vi "GA Get Gear Event.vi"(7 "pStartPara1":dbl, 8 "error in (no error)":errorcluster caption="错误输入（无错误）", 9 "pStartPara0":dbl, 10 "pEvent":i16, 11 "nAxisNum":i16) -> (0 "error out":errorcluster caption="错误输出", 1 "pStartPara0 out":dbl, 2 "pEvent out":i16, 3 "function return":i32, 5 "pStartPara1 out":dbl)   [LabVIEW 2015, in "GAS.lvlib"]
doc: "extern \"C\" __declspec(dllimport) int GA_GetGearEvent(short nAxisNum,short *pEvent,double *pStartPara0,double *pStartPara1);"
uses:
  <userlib>/BP_GAS/GAS.lvlib
  <userlib>/BP_GAS/GAS.dll
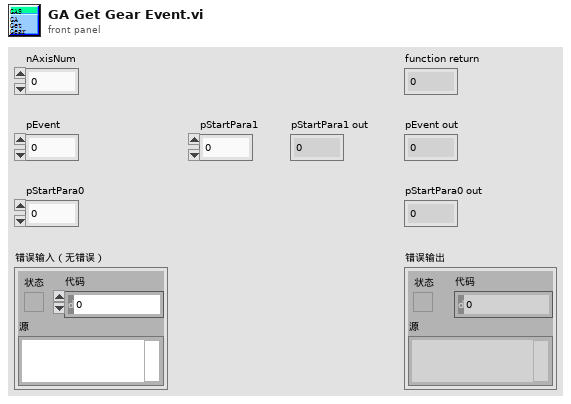
[diagram p1: front panel]
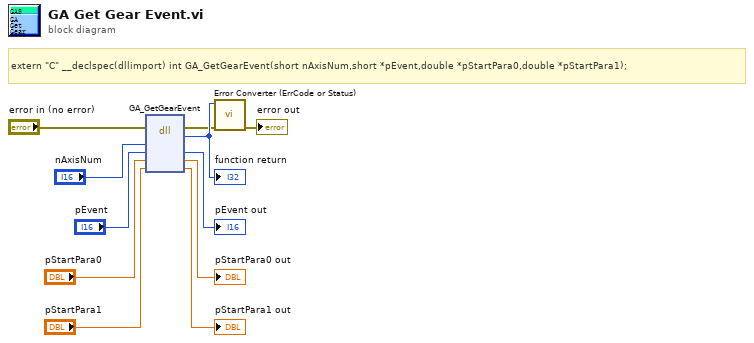
[diagram p0: block diagram]
diagram:
  # "extern \"C\" __declspec(dllimport) int GA_GetGearEvent(short nAxisNum,short *pEvent,double *pStartPara0,double *pStartPara1);"
  n1 = dll-call lib="E:/Program Files (x86)/National Instruments/LabVIEW 2015/user.lib/BP_GAS/GAS.*" fn="GA_GetGearEvent"(error in="error in (no error)", "nAxisNum"="nAxisNum", "pEvent"="pEvent", "pStartPara0"="pStartPara0", "pStartPara1"="pStartPara1") -> (error out=w2:errorcluster, w11:i32, "pEvent"=→"pEvent out":i16, "pStartPara0"=→"pStartPara0 out":dbl, "pStartPara1"=→"pStartPara1 out":dbl)  [unwired: 3 in, 1 out]
  "function return" <- w11
  n2 = call "Error Converter (ErrCode or Status).vi"("error in (no error)"=w2, "error code"=w11) -> ("error out"=→"error out":errorcluster)  [unwired: 9 in]
